vi "PwrM process info.vi"(8 "Name":string="Unknown", 9 "PWR info cluster":T1, 10 "Timestamp":timestamp, 11 "UPS in":T2 {"Last update" format="%<%H:%M:%S>T"}) -> (3 "UPS out":T2 {"Last update" format="%<%H:%M:%S>T"})   [LabVIEW 2024, in "Power monitor.lvlib"]
uses:
  Power monitor.lvlib
  PwrM status.ctl
  .net PowerModeChanged/dotNET PowerModeChanged.llb/SystemPowerStatus.ctl
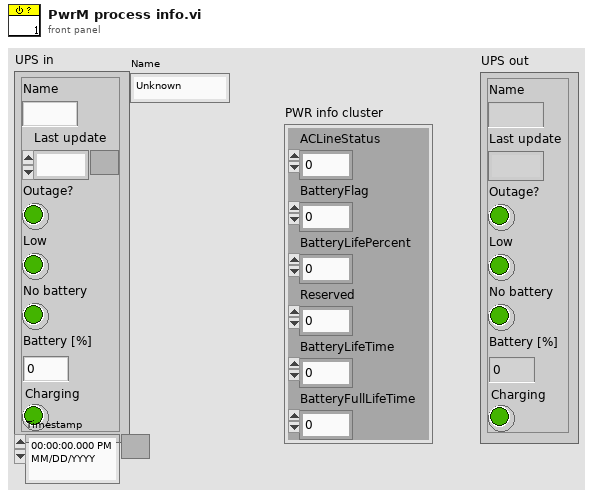
[diagram p1: front panel]
types:
  T1 = typedef "SystemPowerStatus.ctl" = cluster{"ACLineStatus":u8, "BatteryFlag":u8, "BatteryLifePercent":u8, "Reserved":u8, "BatteryLifeTime":i32, "BatteryFullLifeTime":i32}
  T2 = typedef "Power monitor.lvlib/PwrM status.ctl" = cluster{"Name":string, "Last update":timestamp, "Outage?":bool, "Low":bool, "No battery":bool, "Battery [%]":u8, "Charging":bool}
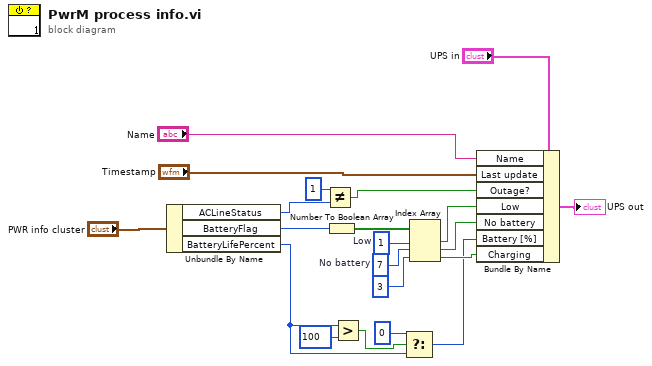
[diagram p0: block diagram]
diagram:
  w20 = 7  # No battery
  w19 = 1  # Low
  n1 = Unbundle By Name("PWR info cluster") -> ("ACLineStatus"=w7:u8, "BatteryFlag"=w13:u8, "BatteryLifePercent"=w10:u8)
  n2 = Not Equal?(x=u8 1, y=w7) -> (x != y?=w6:bool)
  n3 = Number To Boolean Array(number=w13) -> (Boolean array=w12:bool[])
  n4 = Greater?(x=w10, y=u8 100) -> (0:w11:bool)
  n5 = Select(t=u8 0, s=w11, f=w10) -> (s? t:f=w2:u8)
  n6 = Index Array(array=w12, index #1=w19, index #2=w20, index #3=3 ("index")) -> (element #1=w5:bool, element #2=w4:bool, element #3=w3:bool)
  n7 = Bundle By Name(cluster="UPS in", "Name"="Name", "Last update"="Timestamp", "Outage?"=w6, "Low"=w5, "No battery"=w4, "Battery [%]"=w2, "Charging"=w3) -> (→"UPS out":T2)
